vi "Set Single Column Param.vi"(8 "error in (no error)":errorcluster, 9 "Params":string, 10 "column index":i32, 11 "DataGridView in":refnum<class "DataGridView.lvclass">) -> (0 "error out":errorcluster, 3 "DataGridView out":refnum<class "DataGridView.lvclass">)   [LabVIEW 2016, in "DataGrid.lvlib" / "DataGridView.lvclass"]
doc: "Set the params of the index-th column\n\nCopyright @ 2017 Fermion Instruments"
uses:
  <userlib>/LabVIEWdotNetDataGrid/source/DataGridView/DataGridView.lvclass
  <userlib>/LabVIEWdotNetDataGrid/source/DataGridView/DataGridView.lvclass/DataGridView.ctl
  System.Windows.Forms
  <userlib>/LabVIEWdotNetDataGrid/source/GridColumn/GridColumn.lvclass/GridColumn.ctl
  <userlib>/LabVIEWdotNetDataGrid/source/GridColumn/Read Params.vi
  <userlib>/LabVIEWdotNetDataGrid/source/GridColumn/Read datatype.vi
  <userlib>/LabVIEWdotNetDataGrid/source/GridColumn/Read Caption.vi
  <userlib>/LabVIEWdotNetDataGrid/source/GridColumn/Read Name.vi
  <userlib>/LabVIEWdotNetDataGrid/source/GridColumn/Read AutoSizeMode.vi
  <userlib>/LabVIEWdotNetDataGrid/source/GridColumn/Read FillWeight.vi
  <userlib>/LabVIEWdotNetDataGrid/source/GridColumn/Read Tooltip.vi
  <userlib>/LabVIEWdotNetDataGrid/source/GridColumn/Read ReadOnly.vi
  <userlib>/LabVIEWdotNetDataGrid/source/GridColumn/GridColumn.lvclass
  <userlib>/LabVIEWdotNetDataGrid/source/DataTable/DataTable.lvclass
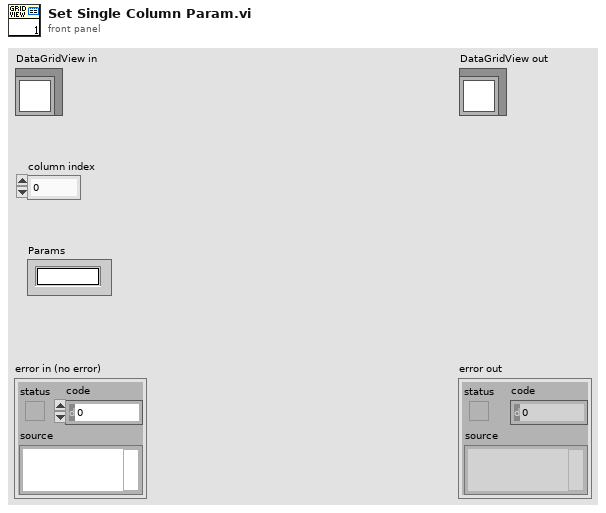
[diagram p1: front panel]
types:
  T1 = typedef "DataGrid.lvlib/GridColumn.lvclass/ColumnType.ctl" = enum16{"string", "image", "check", "numeric", "timestamp", "button", "combo", "link"}
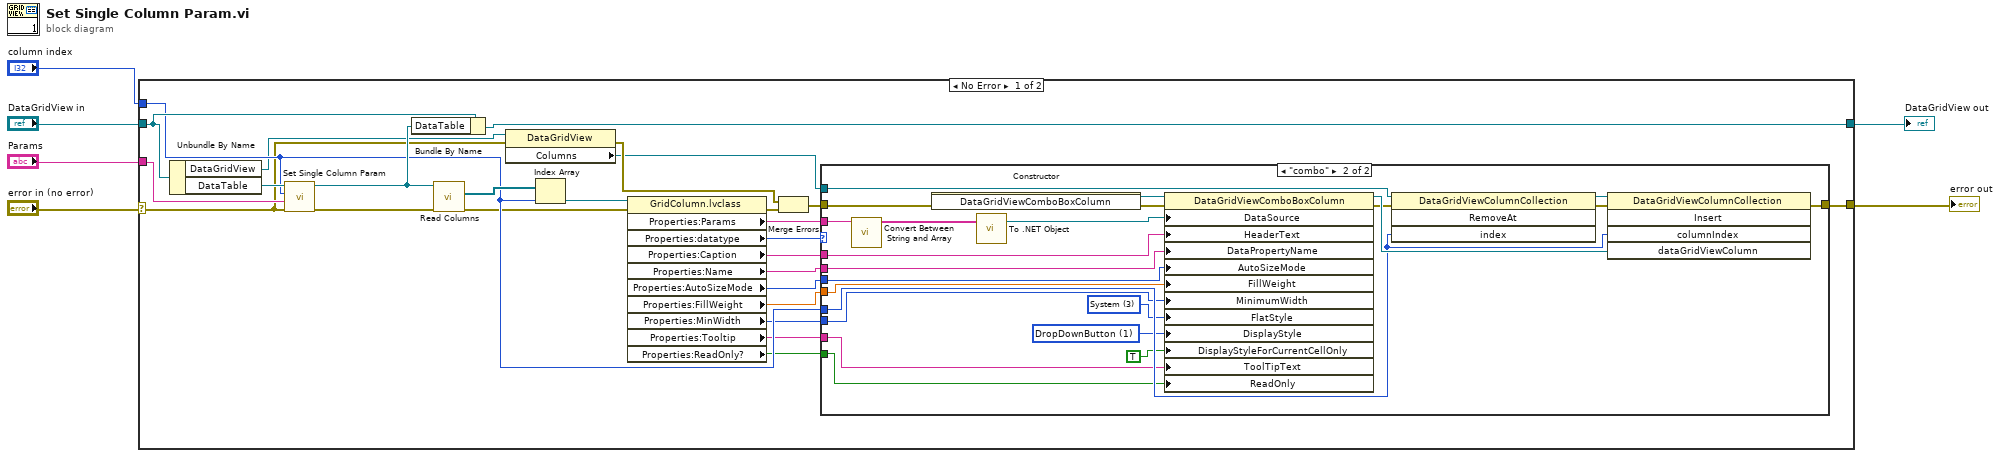
[diagram p0: block diagram]
diagram:
  n1 = case shown="No Error" "error in (no error)" {
    selector: "error in (no error)" -> [w18 w58]
    tunnel: [w19 w58] -> w5
    tunnel: [w30 w57] -> w3
    tunnel: "DataGridView in" -> [w29 w57]
    tunnel: "column index" -> [w23 _]
    tunnel: "Params" -> [w31 _]
    frame No Error {
      n2 = Unbundle By Name(w29) -> ("DataGridView"=w15:refnum<k24>, "DataTable"=w32:refnum<class "DataTable.lvclass">)
      n3 = call <userlib>:"Set Single Column Param.vi"("error in (no error)"=w18, "Params"=w31, "column index"=w23, "DataTable in"=w32) -> ("error out"=w22:errorcluster, "DataTable out"=w28:refnum<class "DataTable.lvclass">)  [unwired: 6 in]
      n4 = Bundle By Name(cluster=w29, "DataTable"=w28) -> (w30:refnum<class "DataGridView.lvclass">)
      n5 = call <userlib>:"Read Columns.vi"("error in (no error)"=w22, "DataTable in"=w28) -> ("error out"=w21:errorcluster, "Columns"=w27:refnum<class "GridColumn.lvclass">[])  [unwired: 7 in, 1 out]
      n6 = property class="DataGridView"(reference=w15, error in=w18) -> (error out=w16:errorcluster, "Columns"=w7:refnum<k24>)  [unwired: 1 out]
      n7 = Index Array(array=w27, index=w23) -> (element=w26:refnum<class "GridColumn.lvclass">)
      n8 = property class="GridColumn.lvclass"(reference=w26, error in=w21) -> (error out=w20:errorcluster, "Properties:Params"=w24:string, "Properties:datatype"=w25:T1, "Properties:Caption"=w14:string, "Properties:Name"=w13:string, "Properties:AutoSizeMode"=w12:i32, "Properties:FillWeight"=w11:sgl, "Properties:MinWidth"=w10:i32, "Properties:Tooltip"=w9:string, "Properties:ReadOnly?"=w8:bool)  [unwired: 1 out]
      n9 = Merge Errors(w16, w20) -> (w17:errorcluster)
      n10 = case shown="\"combo\"" w25 {
        tunnel: w7 -> [_ w54]
        tunnel: [w33 w45] -> w19
        tunnel: w23 -> [_ w46]
        tunnel: w24 -> [_ w47]
        tunnel: w17 -> [w33 w44]
        tunnel: w14 -> [_ w43]
        tunnel: w13 -> [_ w42]
        tunnel: w12 -> [_ w41]
        tunnel: w11 -> [_ w40]
        tunnel: w10 -> [_ w39]
        tunnel: w9 -> [_ w35]
        tunnel: w8 -> [_ w34]
        frame Default {
        }
        frame "combo" {
          w37 = 1 items=["ComboBox", "DropDownButton", "Nothing"] ("DisplayStyle")
          w38 = 3 items=["Flat", "Popup", "Standard", "System"] ("FlatStyle")
          n11 = call <userlib>:"Convert Between String and Array.vi"("String"=w47) -> ("String Array"=w48:string[])  [unwired: 9 in, 1 out]
          n12 = constructor class="DataGridViewComboBoxColumn"(error in=w44) -> (reference out=w56:refnum<k24>, error out=w55:errorcluster)  [unwired: 2 in, 1 out]
          n13 = call <vilib>:"To .NET Object.vi"("anything"=w48) -> (".NET object"=w50:refnum<k24>)  [unwired: 1 in, 1 out]
          n14 = property class="DataGridViewComboBoxColumn"(reference=w56, error in=w55, "DataSource"=w50, "HeaderText"=w43, "DataPropertyName"=w42, "AutoSizeMode"=w41, "FillWeight"=w40, "MinimumWidth"=w39, "FlatStyle"=w38, "DisplayStyle"=w37, "DisplayStyleForCurrentCellOnly"=TRUE, "ToolTipText"=w35, "ReadOnly"=w34) -> (reference out=w51:refnum<k24>, error out=w49:errorcluster)
          n15 = invoke class="DataGridViewColumnCollection" method="RemoveAt"(reference=w54, error in=w49, "index"=w46) -> (reference out=w52:refnum<k24>, error out=w53:errorcluster)  [unwired: 1 in, 2 out]
          n16 = invoke class="DataGridViewColumnCollection" method="Insert"(reference=w52, error in=w53, "columnIndex"=w46, "dataGridViewColumn"=w51) -> (error out=w45:errorcluster)  [unwired: 1 in, 4 out]
        }
      }
    }
    frame Error {
    }
  }
  "error out" <- w5
  "DataGridView out" <- w3
